vi "Strip Tags.vi"(7 "Description in":string) -> (8 "Description out":string)   [LabVIEW 2016]
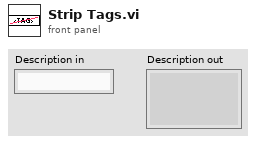
[diagram p1: front panel]
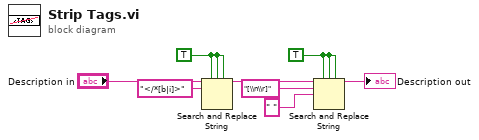
[diagram p0: block diagram]
diagram:
  w1 = TRUE ("replace all? (F)")
  w6 = TRUE ("replace all? (F)")
  n1 = Search and Replace String(replace all?=w6, case sensitive?=w6, multiline?=w6, input string="Description in", search string="</*[b|i]>") -> (result string=w5:string)  [unwired: 3 in, 3 out]
  n2 = Search and Replace String(replace all?=w1, case sensitive?=w1, multiline?=w1, input string=w5, search string="[\\n\\r]", replace string=" " ("replace string (\"\")")) -> (result string=→"Description out":string)  [unwired: 2 in, 3 out]
